vi "例程55-TCP服务端.vi"() -> ()   [LabVIEW 2016]
uses:
  <vilib>/measure/NI_MABase.lvlib
panel:
  out "波形图":waveform(dbl)(graph)={"t0"=timestamp(9142.0 s since 1904-01-01), "dt"=0.001, "Y"=array[1000 elements]}
  out "连接数":i32
  in  "停止":bool
  out "数组":refnum<k5>[](array[refnum])
  out "日期时间":string="2018-11-13 16:34:52"
  out "port":u16=5000 caption="端口"
  in  "amplitude":dbl=1.0 caption="幅值" format="%0.2p"
  in  "signal type":T1(ring)=enum."Sawtooth Wave" caption="信号类型"
  in  "frequency":dbl=2.0 caption="频率" format="%0.2p"
  # "TCP服务端"
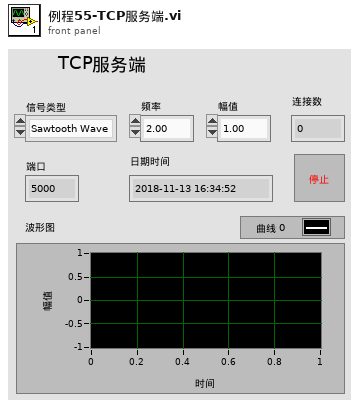
[diagram p1: front panel]
types:
  T1 = enum16{"Sine Wave", "Triangle Wave", "Square Wave", "Sawtooth Wave"}
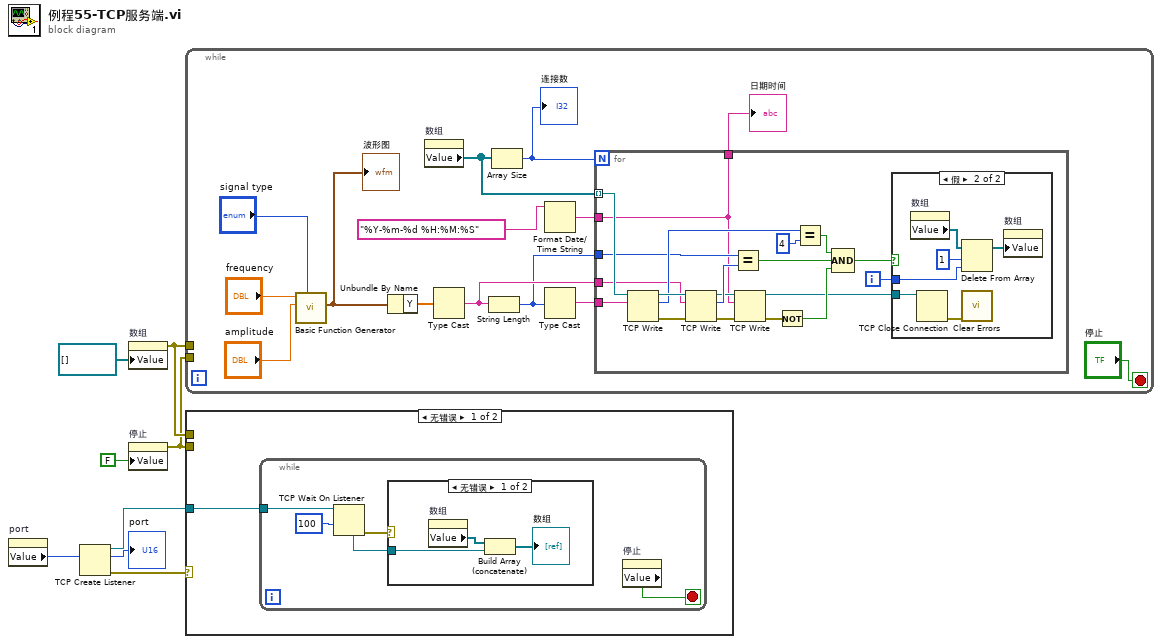
[diagram p0: block diagram]
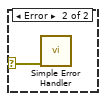
[diagram p4: hidden frame]
diagram:
  n1 = property on="port" class="DigNum (严格)"() -> ("Value"=w6:u16)  [unwired: 2 in, 2 out]
  n2 = TCP Create Listener(10:w6) -> (0:w5:errorcluster, 2:→"port":u16, 3:w8:refnum<k5>)  [unwired: 4 in]
  n3 = property on="数组" class="Arr (严格)"("Value"=refnum<k5>[] [] ("数组")) -> (error out=w3:errorcluster)  [unwired: 2 in, 1 out]
  n4 = property on="停止" class="Bool (严格)"("Value"=FALSE ("停止")) -> (error out=w1:errorcluster)  [unwired: 2 in, 1 out]
  n5 = while {
    tunnel: w3 -> [_]
    tunnel: w1 -> [_]
    stop <- "停止" stop-if-true
    n6 = call <vilib>:"Basic Function Generator.vi"("signal type"="signal type", "amplitude"="amplitude", "frequency"="frequency") -> ("signal out"=w16:waveform(dbl))  [unwired: 6 in, 2 out]
    "波形图" <- w16
    n7 = Unbundle By Name(w16) -> ("Y"=w17:dbl[])
    n8 = property on="数组" class="Arr (严格)"() -> ("Value"=w18:refnum<k5>[])  [unwired: 2 in, 2 out]
    n9 = Type Cast(x=w17) -> (*(type *) &x=w14:string)  [unwired: 1 in]
    n10 = String Length(string=w14) -> (length=w13:i32)
    n11 = Array Size(array=w18) -> (size(s)=w12:i32)
    "连接数" <- w12
    n12 = Format Date/Time String(time format string (%c)="%Y-%m-%d %H:%M:%S" ("时间格式字符串(%c)")) -> (date/time string=w11:string)  [unwired: 2 in]
    n13 = Type Cast(x=w13) -> (*(type *) &x=w15:string)  [unwired: 1 in]
    n14 = for {
      N: w12 -> [_]
      tunnel: w18 -> [w27] mode=indexing
      tunnel: w15 -> [w26]
      tunnel: w14 -> [w25]
      tunnel: w13 -> [w24]
      tunnel: w11 -> [w23]
      tunnel: [w23] -> w10
      i -> [w28]
      n15 = TCP Write(connection ID=w27, data in=w26) -> (connection ID out=w41:refnum<k5>, bytes written=w40:i32, error out=w33:errorcluster)  [unwired: 2 in]
      n16 = TCP Write(connection ID=w41, data in=w25, error in (no error)=w33) -> (connection ID out=w35:refnum<k5>, bytes written=w36:i32, error out=w34:errorcluster)  [unwired: 1 in]
      n17 = Equal?(x=w24, y=w36) -> (x = y?=w37:bool)
      n18 = TCP Write(connection ID=w35, data in=w23, error in (no error)=w34) -> (connection ID out=w29:refnum<k5>, error out=w31:errorcluster)  [unwired: 1 in, 1 out]
      n19 = Not(x=w31) -> (.not. x?=w32:bool)
      n20 = Equal?(x=w40, y=4) -> (x = y?=w38:bool)
      n21 = Compound Arithmetic op=AND ("复合运算")(w38, w37, w32) -> (w30:bool)
      n22 = case shown="假" w30 {
        tunnel: w29 -> [_ w47]
        tunnel: w28 -> [_ w43]
        frame True {
        }
        frame False, Default {
          n23 = property on="数组" class="Arr (严格)"() -> ("Value"=w45:refnum<k5>[])  [unwired: 2 in, 2 out]
          n24 = TCP Close Connection(connection ID=w47) -> (error out=w42:errorcluster)  [unwired: 2 in, 1 out]
          n25 = Delete From Array(array=w45, length=1 ("长度"), index=w43) -> (array with subset deleted=w46:refnum<k5>[])  [unwired: 1 out]
          n26 = call <vilib>:"Clear Errors.vi"("error in (no error)"=w42) -> ()  [unwired: 5 in, 2 out]
          n27 = property on="数组" class="Arr (严格)"("Value"=w46) -> ()  [unwired: 2 in, 2 out]
        }
      }
    }
    "日期时间" <- w10
  }
  n28 = case shown="无错误" w5 {
    selector: w5 -> [_ w57]
    tunnel: w8 -> [w48 _]
    tunnel: w3 -> [_ _]
    tunnel: w1 -> [_ _]
    frame No Error {
      n29 = while {
        tunnel: w48 -> [w53]
        stop <- w50 stop-if-true
        n30 = TCP Wait On Listener(9:100 ("超时毫秒（一直等待:-1）"), 11:w53) -> (0:w52:errorcluster, 4:w51:refnum<k5>)  [unwired: 2 in, 3 out]
        n31 = case shown="无错误" w52 {
          tunnel: w51 -> [w56 _]
          frame No Error {
            n32 = property on="数组" class="Arr (严格)"() -> ("Value"=w54:refnum<k5>[])  [unwired: 2 in, 2 out]
            n33 = Build Array (concatenate)(w54, w56) -> (→"数组":refnum<k5>[])
          }
          frame Error {
          }
        }
        n34 = property on="停止" class="Bool (严格)"() -> ("Value"=w50:bool)  [unwired: 2 in, 2 out]
      }
    }
    frame Error {
      n35 = call <vilib>:"Simple Error Handler.vi"("error in (no error)"=w57) -> ()  [unwired: 4 in, 5 out]
    }
  }
